vi "UnbindEvent.vi"(0 "Event":refnum<event-registration>) -> ()   [LabVIEW 2014]
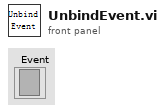
[diagram p1: front panel]
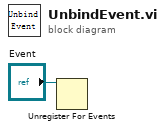
[diagram p0: block diagram]
diagram:
  n1 = Unregister For Events(event registration refnum="Event") -> ()  [unwired: 1 in, 1 out]
